vi "mix_floats.vi"(1 "y":dbl, 2 "alpha":dbl, 3 "x":dbl) -> (0 "alpha * x + (1-alpha) * y":dbl)   [LabVIEW 2010]
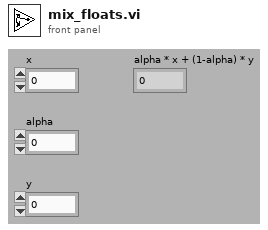
[diagram p1: front panel]
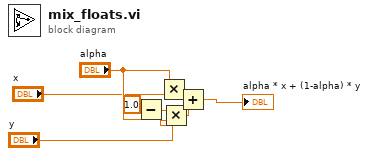
[diagram p0: block diagram]
diagram:
  n1 = Subtract(x=1.0, y="alpha") -> (x-y=w6:dbl)
  n2 = Multiply(x="alpha", y="x") -> (x*y=w2:dbl)
  n3 = Multiply(x=w6, y="y") -> (x*y=w7:dbl)
  n4 = Add(x=w2, y=w7) -> (x+y=→"alpha * x + (1-alpha) * y":dbl)
